vi "robotgyro.vi"(10 "Reset Zero Position":bool, 11 "GyroDevRef in":T1) -> (0 "error out":errorcluster, 2 "GyroDevRef out":T1, 3 "Angle":dbl(knob) scale=0.0..360.0)   [LabVIEW 2011]
uses:
  <vilib>/Rock Robotics/WPI/Gyro/WPI_GyroDevRef.ctl
  <vilib>/Rock Robotics/SystemInterfaces/Typedef/FPGA_TypedefAnalogModule.ctl
  <vilib>/Rock Robotics/SystemInterfaces/AI/FPGA_AIChannel.ctl
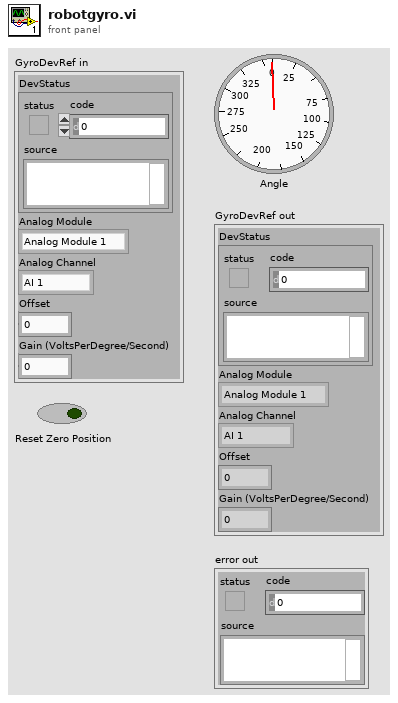
[diagram p1: front panel]
types:
  T1 = typedef "WPI_GyroDevRef.ctl" = cluster{"DevStatus":errorcluster, "Analog Module":T2, "Analog Channel":T3, "Offset":dbl, "Gain (VoltsPerDegree/Second)":dbl}
  T2 = typedef "FPGA_TypedefAnalogModule.ctl" = enum16{"Analog Module 1", "Analog Module 2"}
  T3 = typedef "FPGA_AIChannel.ctl" = enum8{"AI 1", "AI 2", "AI 3", "AI 4", "AI 5", "AI 6", "AI 7", "AI 8", "Invalid"}
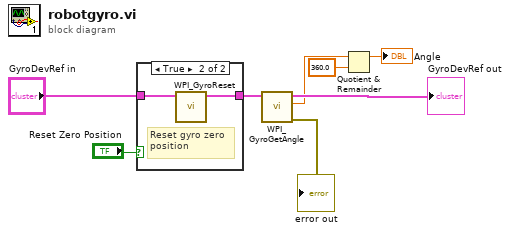
[diagram p0: block diagram]
diagram:
  n1 = case shown="True" "Reset Zero Position" {
    tunnel: "GyroDevRef in" -> [w9 w11]
    tunnel: [w9 w10] -> w3
    frame False {
    }
    frame True {
      # "Reset gyro zero \nposition"
      n2 = call <vilib>:"WPI_GyroReset.vi"("GyroDevRef"=w11) -> ("GyroDevRef"=w10:T1)  [unwired: 10 out]
    }
  }
  n3 = call <vilib>:"WPI_GyroGetAngle.vi"("GyroDevRef"=w3) -> ("error out"=→"error out":errorcluster, "Angle"=w4:dbl, "GyroDevRef"=→"GyroDevRef out":T1)  [unwired: 1 in, 7 out]
  n4 = Quotient & Remainder(x=w4, y=360.0) -> (x-y*floor(x/y)=→"Angle":dbl)  [unwired: 1 out]
